vi "PID -- read interpolate.vi"(0 "sweep folder path":path, 2 "ctl PID file IN":T1, 5 "length":i32, 8 "default":dbl, 9 "temperature":dbl) -> (11 "header":string[](array[string]), 14 "sweep folder path out":path, 16 "PID freq":dbl[](array[numeric]), 17 "PID OK !":bool, 18 "Length OK !":bool, 19 "length out":i32)   [LabVIEW 2015]
uses:
  ctl -- name dispatcher -- action.ctl
  next chunk read-write PID -- action.ctl
  file -- 9w path.vi
  array -- find index - real.vi
  array -- interpolate -- i.vi
  Q -- check range -- i -- real.vi
  Q - not nan -- real.vi
  <vilib>/gmath/function.llb/Binomial Coefficient.vi
  <vilib>/Utility/file.llb/Write To Spreadsheet File.vi
  <vilib>/Utility/file.llb/Write To Spreadsheet File (string).vi
  <vilib>/Utility/libraryn.llb/Check if File or Folder Exists.vi
  parse -- get list of matches -- numbers.vi
  parse -- find first line.vi
  file -- read list of lines.vi
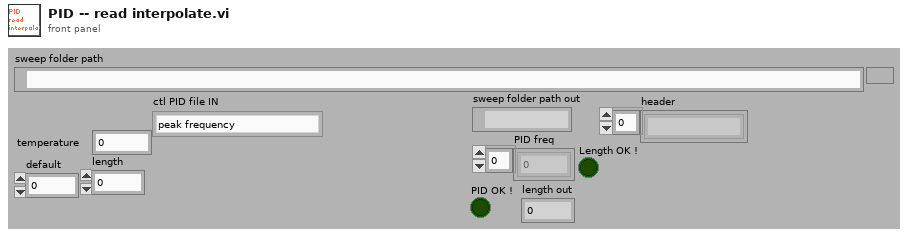
[diagram p1: front panel]
types:
  T1 = typedef "ctl -- name dispatcher -- action.ctl" = enum16{"peak frequency", "peak frequency DUMP", "peak gamma DUMP", "peak gamma", "peak frequency TEST", "peak gamma TEST", "ultrasonic power", "time in gamma", "set temperature ", "set temperature timer", "peak default gamma", "last scan file", "peak freq gamma TEST", "peak NAMES", "errors", "P_I_D", "P", "I", "D", "power vs time", "power vs time TIMER", "void", "power log", "set temperature - SINE", "itc ltc log", "peak - time in gamma"}
  T2 = typedef "next chunk read-write PID -- action.ctl" = enum16{"read", "interpolate", "append col", "write", "write PID col", "append PID col", "interpolate - bezier"}
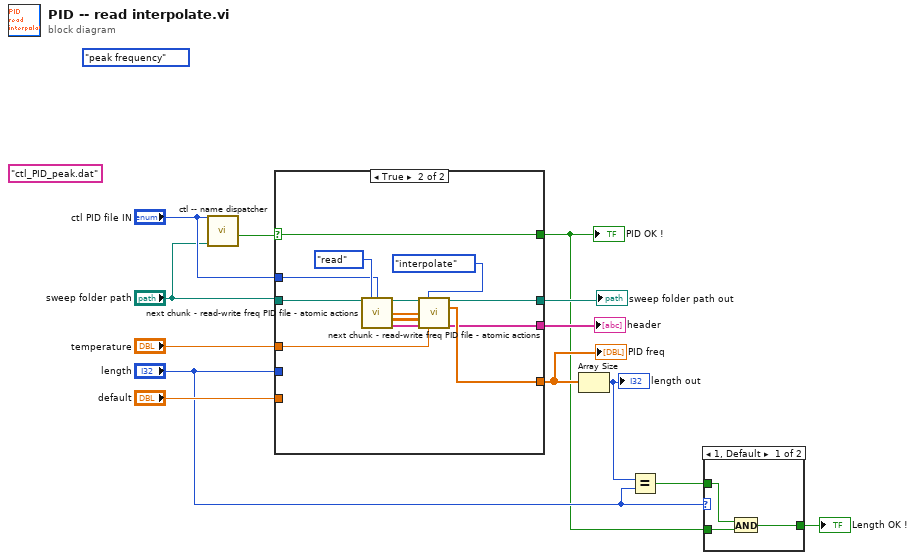
[diagram p0: block diagram]
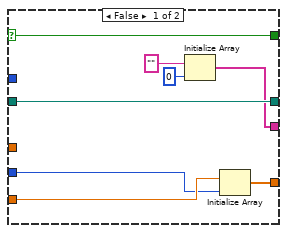
[diagram p3: hidden frame]
diagram:
  (unwired) ctl_--_name_dispatcher_--_action."peak frequency" ("ctl PID file IN")
  (unwired) "ctl_PID_peak.dat" ("freq PID file OUT")
  n1 = call "ctl -- name dispatcher.vi"("sweep folder path"="sweep folder path", "ctl name dispatch"="ctl PID file IN") -> ("file or folder exists?"=w6:bool)  [unwired: 7 in, 2 out]
  n2 = case shown="True" w6 {
    selector: w6 -> [w20 w25]
    tunnel: "sweep folder path" -> [w21 w30]
    tunnel: [w21 w28] -> w13
    tunnel: "temperature" -> [_ w27]
    tunnel: [w18 w26] -> w10
    tunnel: [w20 w25] -> w2
    tunnel: "default" -> [w19 _]
    tunnel: "length" -> [w16 _]
    tunnel: [w17 w24] -> w9
    tunnel: "ctl PID file IN" -> [_ w23]
    frame False {
      n3 = Initialize Array("" ("freq PID file OUT"), 0 ("dimension size")) -> (w17:string[])
      n4 = Initialize Array(w19, w16) -> (w18:dbl[])
    }
    frame True {
      n5 = call "next chunk - read-write freq PID file - atomic actions .vi"("sweep folder path"=w30, "PID action"=next_chunk_read-write_PID_--_action."read", "ctl kind IN"=w23) -> ("sweep folder path out"=w33:path, "temperatures"=w31:dbl[], "frequencies"=w32:dbl[][], "header"=w22:string[])  [unwired: 8 in, 1 out]
      n6 = call "next chunk - read-write freq PID file - atomic actions .vi"("sweep folder path"=w33, "PID action"=next_chunk_read-write_PID_--_action."interpolate", "temperatures IN"=w31, "frequencies IN"=w32, "header IN"=w22, "temperature"=w27) -> ("sweep folder path out"=w28:path, "PID freq"=w26:dbl[], "header"=w24:string[])  [unwired: 5 in, 2 out]
    }
  }
  "sweep folder path out" <- w13
  "PID freq" <- w10
  "PID OK !" <- w2
  "header" <- w9
  n7 = Array Size(array=w10) -> (size(s)=w5:i32)
  "length out" <- w5
  n8 = Equal?(x=w5, y="length") -> (x = y?=w1:bool)
  n9 = case shown="1, Default" "length" {
    tunnel: [w35 w38] -> w3
    tunnel: w2 -> [w37 w38]
    tunnel: w1 -> [w36 _]
    frame 1, Default {
      n10 = And(x=w36, y=w37) -> (x .and. y?=w35:bool)
    }
    frame 0 {
    }
  }
  "Length OK !" <- w3
